vi "IsROIChange.vi"(9 "InputData":u32[](array[numeric]), 11 "ROI":T1) -> (1 "OutputData":u32[](array[numeric]), 3 "Change?":bool)   [LabVIEW 2015]
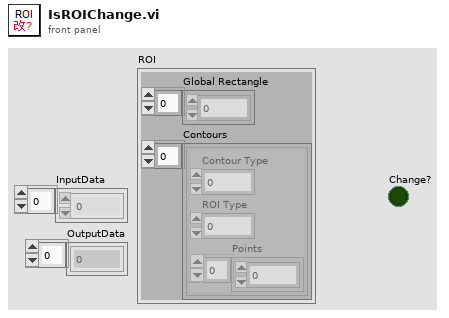
[diagram p1: front panel]
types:
  T1 = cluster{"Global Rectangle":i32[], "Contours":cluster{"Contour Type":u32, "ROI Type":u32, "Points":i32[]}[]}
  T2 = cluster{"Contour Type":u32, "ROI Type":u32, "Points":i32[]}[]
  T3 = cluster{"Contour Type":u32, "ROI Type":u32, "Points":i32[]}
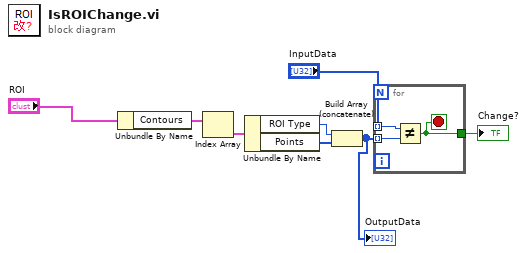
[diagram p0: block diagram]
diagram:
  n1 = Unbundle By Name("ROI") -> ("Contours"=w7:T2)
  n2 = Index Array(array=w7) -> (element=w8:T3)  [unwired: 1 in]
  n3 = Unbundle By Name(w8) -> ("ROI Type"=w6:u32, "Points"=w5:i32[])
  n4 = Build Array (concatenate)(w6, w5) -> (w1:u32[])
  "OutputData" <- w1
  n5 = for {
    tunnel: "InputData" -> [w11] mode=indexing
    tunnel: w1 -> [w10] mode=indexing
    tunnel: [w9] -> w3
    stop <- w9 stop-if-true
    n6 = Not Equal?(x=w11, y=w10) -> (x != y?=w9:bool)
  }
  "Change?" <- w3
